vi "Unpack Control Mouse Down.vi"(11 "ControlMouseDownMsg":refnum<class "ControlMouseDownMsg.lvclass">) -> (0 "Button":u16, 1 "Coords":T2, 2 "Time":u32, 3 "Name":string, 4 "Mods":cluster{"Double Click":bool, "Menu Key":bool}, 6 "PlatMods":T1)   [LabVIEW 2015, in "ActorAutoRegistration.lvlib" / "ControlMouseDownMsg.lvclass"]
uses:
  ControlMouseDownMsg.lvclass
  <vilib>/Utility/miscctls.llb/LVPoint32TypeDef.ctl
  ControlMouseDownMsg.lvclass/ControlMouseDownMsg.ctl
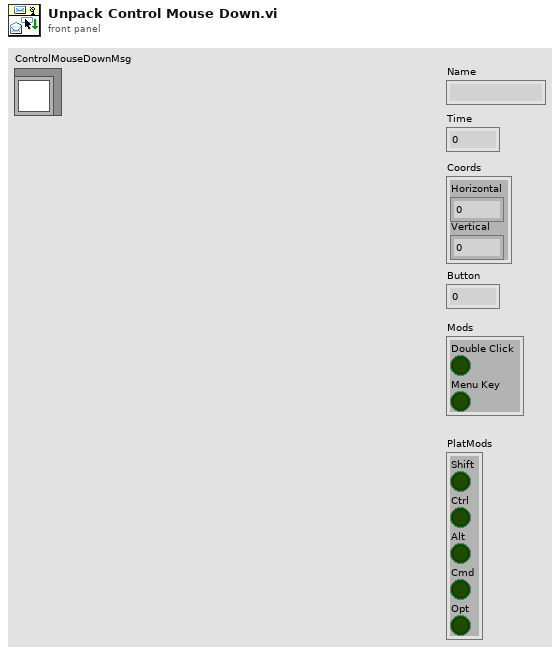
[diagram p1: front panel]
types:
  T1 = cluster{"Shift":bool, "Ctrl":bool, "Alt":bool, "Cmd":bool, "Opt":bool}
  T2 = typedef "LVPoint32TypeDef.ctl" = cluster{"Horizontal":i32, "Vertical":i32}
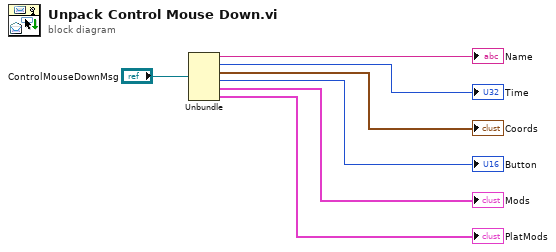
[diagram p0: block diagram]
diagram:
  n1 = Unbundle("ControlMouseDownMsg") -> (→"Name":string, →"Time":u32, →"Coords":T2, →"Button":u16, →"Mods":cluster{"Double Click":bool, "Menu Key":bool}, →"PlatMods":T1)
